vi "Compute Gyro Turn.vi"(8 "error in (no error)":errorcluster, 11 "Turn? Right Positive.":dbl) -> (0 "error out":errorcluster, 2 "Right Drive":dbl, 3 "Left drive":dbl, 5 "done":bool)   [LabVIEW 2017]
uses:
  Robot Global Data.vi
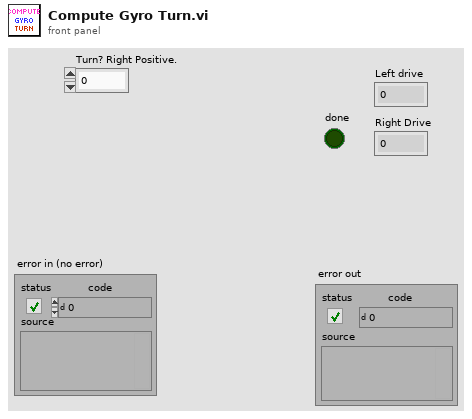
[diagram p1: front panel]
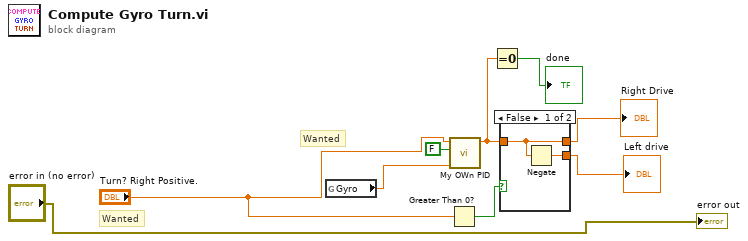
[diagram p0: block diagram]
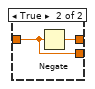
[diagram p2: hidden frame]
diagram:
  # "Wanted"
  # "Wanted"
  n1 = global read "Robot Global Data.vi" "Gyro"() -> (w5:dbl)
  n2 = Greater Than 0?(x="Turn? Right Positive.") -> (x > 0?=w9:bool)
  n3 = call "My OWn PID.vi"("Current Input"=w5, "Encoders (t) gyro (f)"=FALSE, "Wanted End"="Turn? Right Positive.") -> ("Output"=w3:dbl)  [unwired: 8 in]
  n4 = Equal To 0?(x=w3) -> (x = 0?=→"done":bool)
  n5 = case shown="False" w9 {
    tunnel: w3 -> [w10 w12]
    tunnel: [w10 w13] -> w7
    tunnel: [w11 w12] -> w8
    frame False {
      n6 = Negate(x=w10) -> (-x=w11:dbl)
    }
    frame True {
      n7 = Negate(x=w12) -> (-x=w13:dbl)
    }
  }
  "Left drive" <- w8
  "Right Drive" <- w7
  "error out" <- "error in (no error)"
